vi "NI_STRING_DATA (SubVI).vi"(11 "Value":bool[](array[boolean])) -> (3 "String":string)   [LabVIEW 2020]
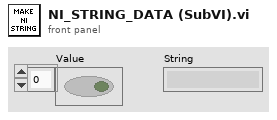
[diagram p1: front panel]
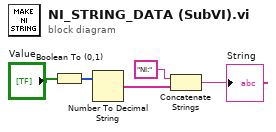
[diagram p0: block diagram]
diagram:
  n1 = Boolean To (0,1)(Boolean="Value") -> (0, 1=w2:i16[])
  n2 = Number To Decimal String(number=w2) -> (decimal integer string=w3:string[])  [unwired: 1 in]
  n3 = Concatenate Strings("NI:" ("string"), w3) -> (→"String":string)
